vi "Kinect Process Image.vi"(0 "Depth Image In":T1, 5 "Distance to Camera Visible":cluster{dbl, dbl}(slide)={0.0, 32768.0} scale=-32768.0..32768.0, 7 "Median Filter Size":i32 min=0 max=7, 9 "Divisor":sgl=1.0 min=0 max=1 step=0.1, 11 "error in (no error)":errorcluster) -> (4 "Image Dst Out":T1, 15 "error out":errorcluster)   [LabVIEW 2011]
uses:
  <vilib>/vision/Image Controls.llb/IMAQ Image.ctl
  <vilib>/vision/NI_Vision_Development_Module.lvlib
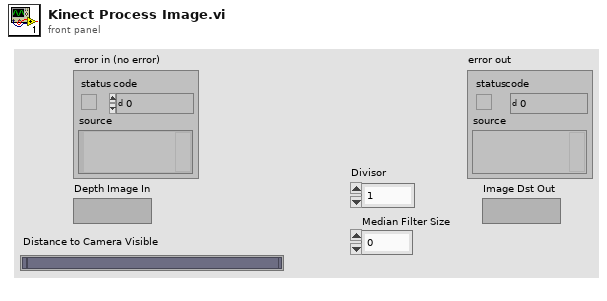
[diagram p1: front panel]
types:
  T1 = typedef "IMAQ Image.ctl" = refnum<image>
  T2 = enum32{"Average", "Min", "Max", "Clear  if < ", "Clear  if < or =", "Clear  if =", "Clear  if > or =", "Clear  if >"}
  T3 = cluster{"Median Filter Size":i32, "Median Filter Size":i32, i32}
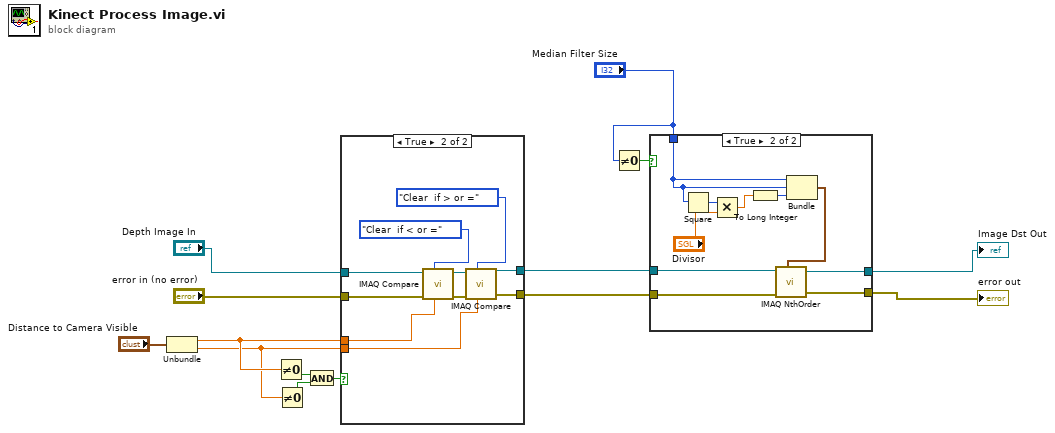
[diagram p0: block diagram]
diagram:
  n1 = Unbundle("Distance to Camera Visible") -> (w3:dbl, w2:dbl)
  n2 = Not Equal To 0?(x=w3) -> (x != 0?=w4:bool)
  n3 = Not Equal To 0?(x=w2) -> (x != 0?=w5:bool)
  n4 = And(x=w4, y=w5) -> (x .and. y?=w1:bool)
  n5 = case shown="True" w1 {
    tunnel: "error in (no error)" -> [w15 w22]
    tunnel: "Depth Image In" -> [w16 w21]
    tunnel: [w16 w20] -> w10
    tunnel: [w15 w19] -> w9
    tunnel: w3 -> [_ w18]
    tunnel: w2 -> [_ w17]
    frame False {
    }
    frame True {
      n6 = call "IMAQ Compare"("Constant"=w18, "Operator"=T2."Clear  if < or =", "error in (no error)"=w22, "Image Src A"=w21) -> ("error out"=w24:errorcluster, "Image Dst Out"=w23:T1)  [unwired: 6 in]
      n7 = call "IMAQ Compare"("Constant"=w17, "Operator"=T2."Clear  if > or =", "error in (no error)"=w24, "Image Src A"=w23) -> ("error out"=w19:errorcluster, "Image Dst Out"=w20:T1)  [unwired: 6 in]
    }
  }
  n8 = Not Equal To 0?(x="Median Filter Size") -> (x != 0?=w7:bool)
  n9 = case shown="True" w7 {
    tunnel: [w28 w36] -> w11
    tunnel: w10 -> [w28 w35]
    tunnel: w9 -> [w27 w34]
    tunnel: [w27 w33] -> w8
    tunnel: "Median Filter Size" -> [_ w32]
    frame False {
    }
    frame True {
      n10 = Square(x=w32) -> (x^2=w31:i32)
      n11 = Multiply(x=w31, y="Divisor") -> (x*y=w29:sgl)
      n12 = To Long Integer(number=w29) -> (32bit integer=w38:i32)
      n13 = Bundle("Median Filter Size"=w32, "Median Filter Size"=w32, w38) -> (w37:T3)  [unwired: 1 in]
      n14 = call "IMAQ NthOrder"("Image Src"=w35, "Size & Order #"=w37, "error in (no error)"=w34) -> ("Image Dst Out"=w36:T1, "error out"=w33:errorcluster)  [unwired: 4 in]
    }
  }
  "error out" <- w8
  "Image Dst Out" <- w11
